vi "Teleop.vi"(10 "Match Info":T1={"Autonomous Elapsed Seconds"=15.277, "TeleOp Elapsed Seconds"=16.177, "Disabled Elapsed Seconds"=3.92, "Visited Autonomous"=TRUE, "Visited TeleOp"=TRUE, "Visited Disabled"=TRUE, "Autonomous Settings"={"Autonomous Style"=enum."Independent", "VI Refnum"=refnum}}, 11 "Call Context":T2=enum."Stop") -> ()   [LabVIEW 2016]
doc: "This VI is called for each TeleOp packet received from the DS where the robot is not disabled. It is often used to read from the joysticks and update I/O or to update setpoints for timed control loops. It should complete and return within 20 milliseconds or it may miss DS packets."
uses:
  <vilib>/Rock Robotics/WPI/DriverStation/WPI_DriverStationDerivedRobotMode.ctl
  <vilib>/Rock Robotics/WPI/DriverStation/WPI_DriverStationMatch Info.ctl
  <vilib>/Rock Robotics/WPI/Utilities/WPI_GetSetVariantRefNum.vi
  Robot Global Data.vi
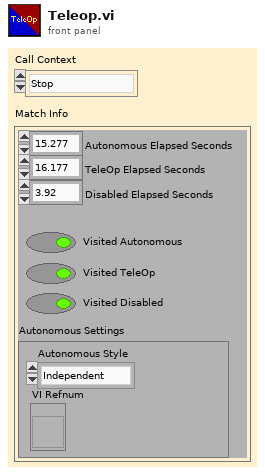
[diagram p1: front panel]
types:
  T1 = typedef "WPI_DriverStationMatch Info.ctl" = cluster{"Autonomous Elapsed Seconds":dbl, "TeleOp Elapsed Seconds":dbl, "Disabled Elapsed Seconds":dbl, "Visited Autonomous":bool, "Visited TeleOp":bool, "Visited Disabled":bool, "Autonomous Settings":cluster{"Autonomous Style":enum16{"Iterative", "Independent"}, "VI Refnum":refnum<vi>}}
  T2 = typedef "WPI_DriverStationDerivedRobotMode.ctl" = enum16{"Init", "Execute", "Stop"}
  T3 = typedef "WPI_JoystickDevRef.ctl" = cluster{"Device":T4}
  T4 = typedef "WPI_JoystickDeviceEnum.ctl" = enum16{"USB 0", "USB 1", "USB 2", "USB 3", "USB 4", "USB 5"}
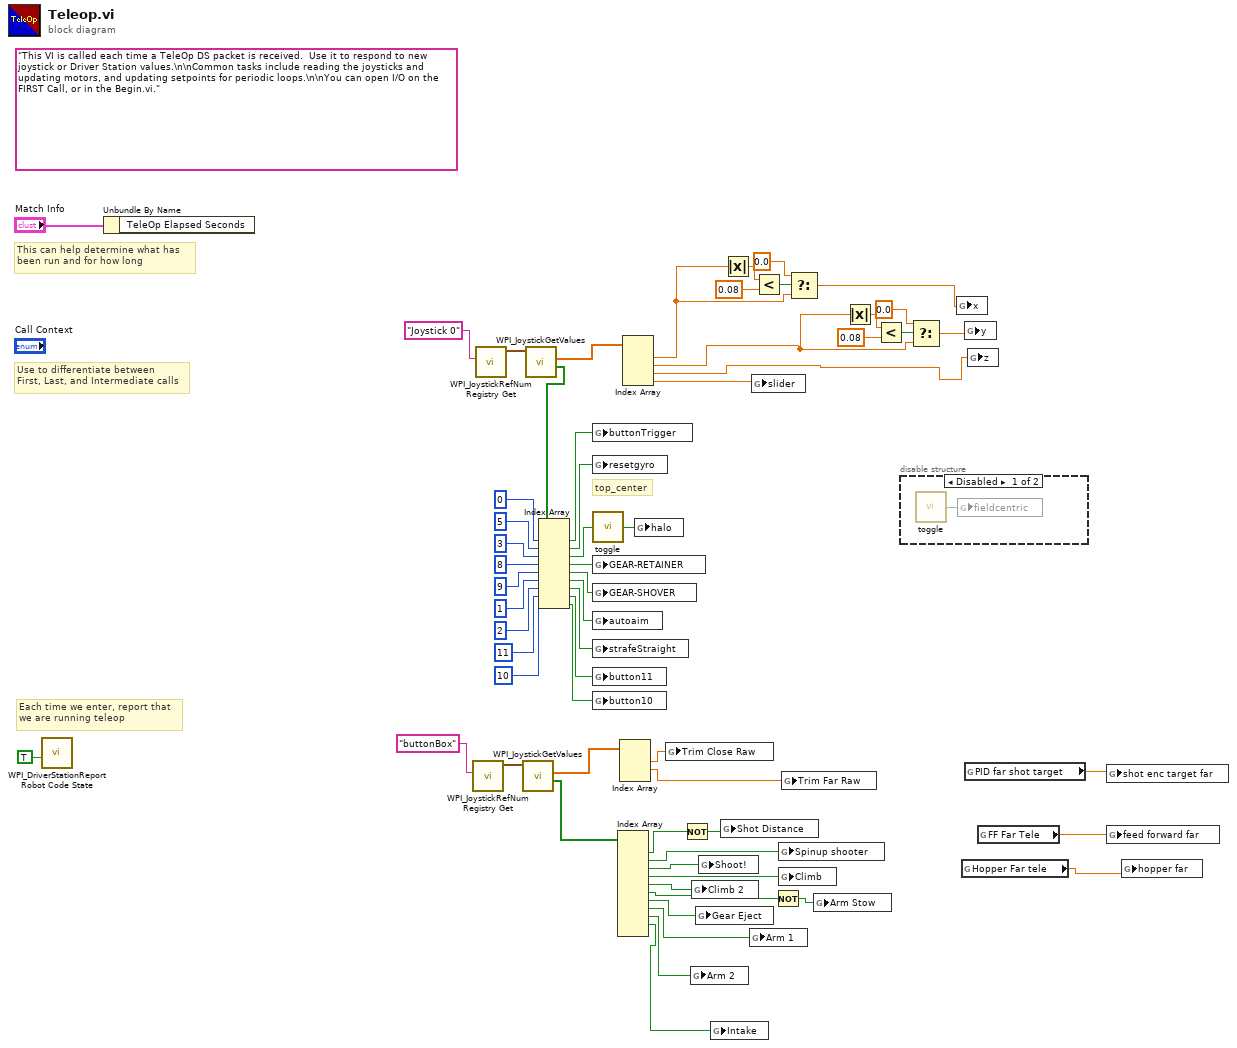
[diagram p0: block diagram]
diagram:
  (unwired) "This VI is called each time a TeleOp DS packet is received.  Use it to respond to new joystick or Driver Station values.\n\nCommon tasks include reading the joysticks and updating motors, and updating setpoints for periodic loops.\n\nYou can open I/O on the FIRST Call, or in the Begin.vi."
  # "top_center"
  # "Each time we enter, report that\nwe are running teleop"
  # "Use to differentiate between\nFirst, Last, and Intermediate calls"
  # "This can help determine what has\nbeen run and for how long"
  n1 = call <vilib>:"WPI_DriverStationReport Robot Code State.vi"("TeleOp"=TRUE ("Autonomous")) -> ()  [unwired: 10 in, 1 out]
  n2 = Unbundle By Name("Match Info") -> ()  [unwired: 1 out]
  n3 = call <vilib>:"WPI_JoystickRefNum Registry Get.vi"("refnum name"="buttonBox") -> ("JoystickDevRef"=w40:T3)  [unwired: 1 in, 9 out]
  n4 = call <vilib>:"WPI_JoystickRefNum Registry Get.vi"("refnum name"="Joystick 0") -> ("JoystickDevRef"=w58:T3)  [unwired: 1 in, 9 out]
  n5 = call <vilib>:"WPI_JoystickGetValues.vi"("JoystickDevRef"=w40) -> ("Buttons"=w38:bool[], "Axes"=w39:dbl[])  [unwired: 6 in, 3 out]
  n6 = call <vilib>:"WPI_JoystickGetValues.vi"("JoystickDevRef"=w58) -> ("Buttons"=w55:bool[], "Axes"=w56:dbl[])  [unwired: 6 in, 3 out]
  n7 = Index Array(array=w55, index #1=0 ("index"), index #2=5 ("index"), index #3=3 ("index"), index #4=8 ("index"), index #5=9 ("index"), index #6=1 ("index"), index #7=2 ("index"), index #8=11 ("index"), index #9=10 ("index")) -> (element #1=w1:bool, element #2=w53:bool, element #3=w52:bool, element #4=w44:bool, element #5=w43:bool, element #6=w21:bool, element #7=w28:bool, element #8=w17:bool, element #9=w10:bool)
  n8 = global write "Robot Global Data.vi" "buttonTrigger"(w1) -> ()
  n9 = global write "Robot Global Data.vi" "resetgyro"(w53) -> ()
  n10 = call "toggle.vi"("Input"=w52) -> ("Output"=w54:bool)
  n11 = global write "Robot Global Data.vi" "GEAR-RETAINER"(w44) -> ()
  n12 = global write "Robot Global Data.vi" "GEAR-SHOVER"(w43) -> ()
  n13 = global write "Robot Global Data.vi" "autoaim"(w21) -> ()
  n14 = global write "Robot Global Data.vi" "strafeStraight"(w28) -> ()
  n15 = global write "Robot Global Data.vi" "button11"(w17) -> ()
  n16 = global write "Robot Global Data.vi" "button10"(w10) -> ()
  n17 = Index Array(array=w38) -> (element #1=w31:bool, element #2=w19:bool, element #3=w37:bool, element #4=w36:bool, element #5=w35:bool, element #6=w16:bool, element #7=w26:bool, element #8=w25:bool, element #9=w24:bool, element #10=w23:bool)  [unwired: 11 in, 1 out]
  n18 = Index Array(array=w39) -> (element #1=w33:dbl, element #2=w34:dbl)  [unwired: 3 in, 1 out]
  n19 = Index Array(array=w56) -> (element #1=w47:dbl, element #2=w3:dbl, element #3=w8:dbl, element #4=w22:dbl)  [unwired: 4 in]
  n20 = global write "Robot Global Data.vi" "halo"(w54) -> ()
  n21 = global write "Robot Global Data.vi" "Trim Close Raw"(w33) -> ()
  n22 = Not(x=w31) -> (.not. x?=w32:bool)
  n23 = global write "Robot Global Data.vi" "Arm 2"(w24) -> ()
  n24 = global write "Robot Global Data.vi" "Climb 2"(w35) -> ()
  n25 = global write "Robot Global Data.vi" "Gear Eject"(w26) -> ()
  n26 = global write "Robot Global Data.vi" "Shoot!"(w37) -> ()
  n27 = global write "Robot Global Data.vi" "Intake"(w23) -> ()
  n28 = global write "Robot Global Data.vi" "Shot Distance"(w32) -> ()
  n29 = Absolute Value(x=w47) -> (abs(x)=w50:dbl)
  n30 = global write "Robot Global Data.vi" "Arm 1"(w25) -> ()
  n31 = global write "Robot Global Data.vi" "slider"(w22) -> ()
  n32 = Less?(x=w50, y=0.08) -> (x < y?=w49:bool)
  n33 = Not(x=w16) -> (.not. x?=w15:bool)
  n34 = global write "Robot Global Data.vi" "Spinup shooter"(w19) -> ()
  n35 = global write "Robot Global Data.vi" "Climb"(w36) -> ()
  n36 = global write "Robot Global Data.vi" "Trim Far Raw"(w34) -> ()
  n37 = Select(t=0.0, s=w49, f=w47) -> (s? t:f=w46:dbl)
  n38 = global write "Robot Global Data.vi" "Arm Stow"(w15) -> ()
  n39 = Absolute Value(x=w3) -> (abs(x)=w6:dbl)
  n40 = Less?(x=w6, y=0.08) -> (x < y?=w5:bool)
  n41 = disable-structure shown="Disabled" {
    frame Disabled {
      n42 = call "toggle.vi"() -> ("Output"=w61:bool)  [unwired: 1 in]
      n43 = global write "Robot Global Data.vi" "fieldcentric"(w61) -> ()
    }
    frame Enabled {
    }
  }
  n44 = Select(t=0.0, s=w5, f=w3) -> (s? t:f=w2:dbl)
  n45 = global write "Robot Global Data.vi" "x"(w46) -> ()
  n46 = global read "Robot Global Data.vi" "Hopper Far tele"() -> (w13:dbl)
  n47 = global write "Robot Global Data.vi" "y"(w2) -> ()
  n48 = global read "Robot Global Data.vi" "PID far shot target"() -> (w9:dbl)
  n49 = global write "Robot Global Data.vi" "z"(w8) -> ()
  n50 = global read "Robot Global Data.vi" "FF Far Tele"() -> (w14:dbl)
  n51 = global write "Robot Global Data.vi" "shot enc target far"(w9) -> ()
  n52 = global write "Robot Global Data.vi" "feed forward far"(w14) -> ()
  n53 = global write "Robot Global Data.vi" "hopper far"(w13) -> ()
